vi "Target volume start.vi"(6 "Pump Direction (0:Infuse)":u16(ring) items=["Infuse", "Withdraw"], 8 "error in (no error)":errorcluster, 9 "Flow Rate (ml/min)":dbl=5.0 format="%#.4f", 10 "Target volume (ml)":dbl=5.0 format="%#.4f", 11 "VISA resource name":refnum<visa-resource-name>) -> (0 "error out":errorcluster, 3 "VISA resource name out":refnum<visa-resource-name>)   [LabVIEW 2017]
uses:
  <instrlib>/Harvard Apparatus PHD Ultra Series/Harvard Apparatus PHD Ultra Series.lvlib
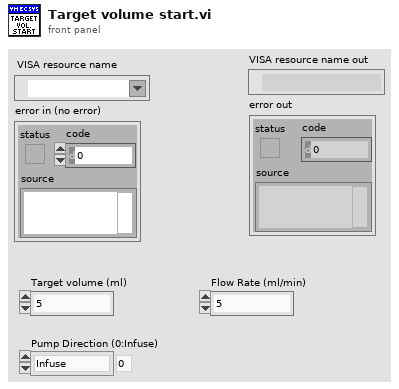
[diagram p1: front panel]
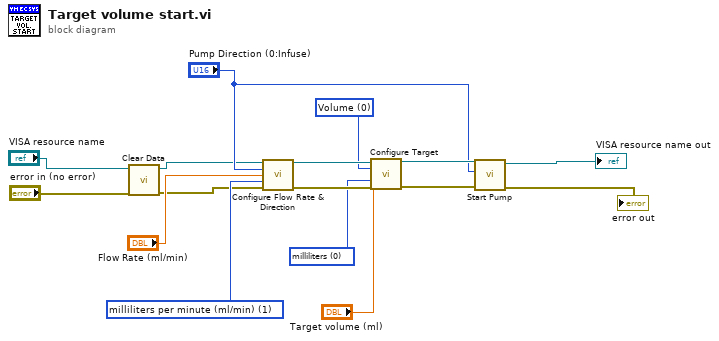
[diagram p0: block diagram]
diagram:
  w5 = u32 1 items=["milliliters per hour (ml/hr)", "milliliters per minute (ml/min)", "milliliters per second (ml/sec)", "microliters per hour (ul/hr)", "microliters per minute (ul/min)", "microliters per second (ul/sec)", "nanoliters per hour (nl/hr)", "nanoliters per minute (nl/min)", "nanoliters per second (nl/sec)", "picoliters per hour (pl/hr)", "picoliters per minute (pl/min)", "picoliters per second (pl/sec)"] ("Flow Rate Units (1:ml/min)")
  w10 = u16 0 items=["Volume", "Time"] ("Target Type (0:Volume)")
  w12 = u16 0 items=["milliliters", "microliters", "nanoliters", "picoliters"] ("Volume Units (0:ml)")
  n1 = call <instrlib>:"Clear Data.vi"("error in (no error)"="error in (no error)", "VISA resource name"="VISA resource name") -> ("error out"=w3:errorcluster, "VISA resource name out"=w4:refnum<visa-resource-name>)  [unwired: 8 in]
  n2 = call <instrlib>:"Configure Flow Rate & Direction.vi"("VISA resource name"=w4, "Pump Direction (0:Infuse)"="Pump Direction (0:Infuse)", "Flow Rate (5.00)"="Flow Rate (ml/min)", "Flow Rate Units (1:ml/min)"=w5, "error in (no error)"=w3) -> ("VISA resource name out"=w16:refnum<visa-resource-name>, "error out"=w14:errorcluster)  [unwired: 9 in]
  n3 = call <instrlib>:"Configure Target.vi"("VISA resource name"=w16, "Target Type (0:Volume)"=w10, "Target Value (5.00)"="Target volume (ml)", "Volume Units (0:ml)"=w12, "error in (no error)"=w14) -> ("VISA resource name out"=w15:refnum<visa-resource-name>, "error out"=w13:errorcluster)  [unwired: 9 in]
  n4 = call <instrlib>:"Start Pump.vi"("error in (no error)"=w13, "Run Direction (0:Infuse)"="Pump Direction (0:Infuse)", "VISA resource name"=w15) -> ("error out"=→"error out":errorcluster, "VISA resource name out"=→"VISA resource name out":refnum<visa-resource-name>)  [unwired: 7 in]
